vi "CRYGet Scale Format Info.vi"(11 "FormatString":string) -> (3 "ScaleFormat":T1)   [LabVIEW 2013]
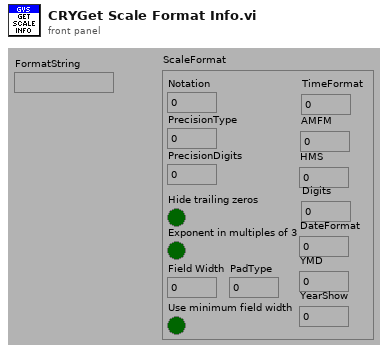
[diagram p1: front panel]
types:
  T1 = cluster{"Notation":i32, "PrecisionType":u16, "PrecisionDigits":u16, "Hide trailing zeros":bool, "Exponent in multiples of 3":bool, "Field Width":u16, "PadType":u16, "Use minimum field width":bool, "TimeFormat":u16, "AMFM":u16, "HMS":u16, "Digits":u16, "DateFormat":u16, "YMD":u16, "YearShow":u16}
  T2 = enum16{"OK", "Yes", "YesNo", "YesNoCancel", "ReplaceAppend"}
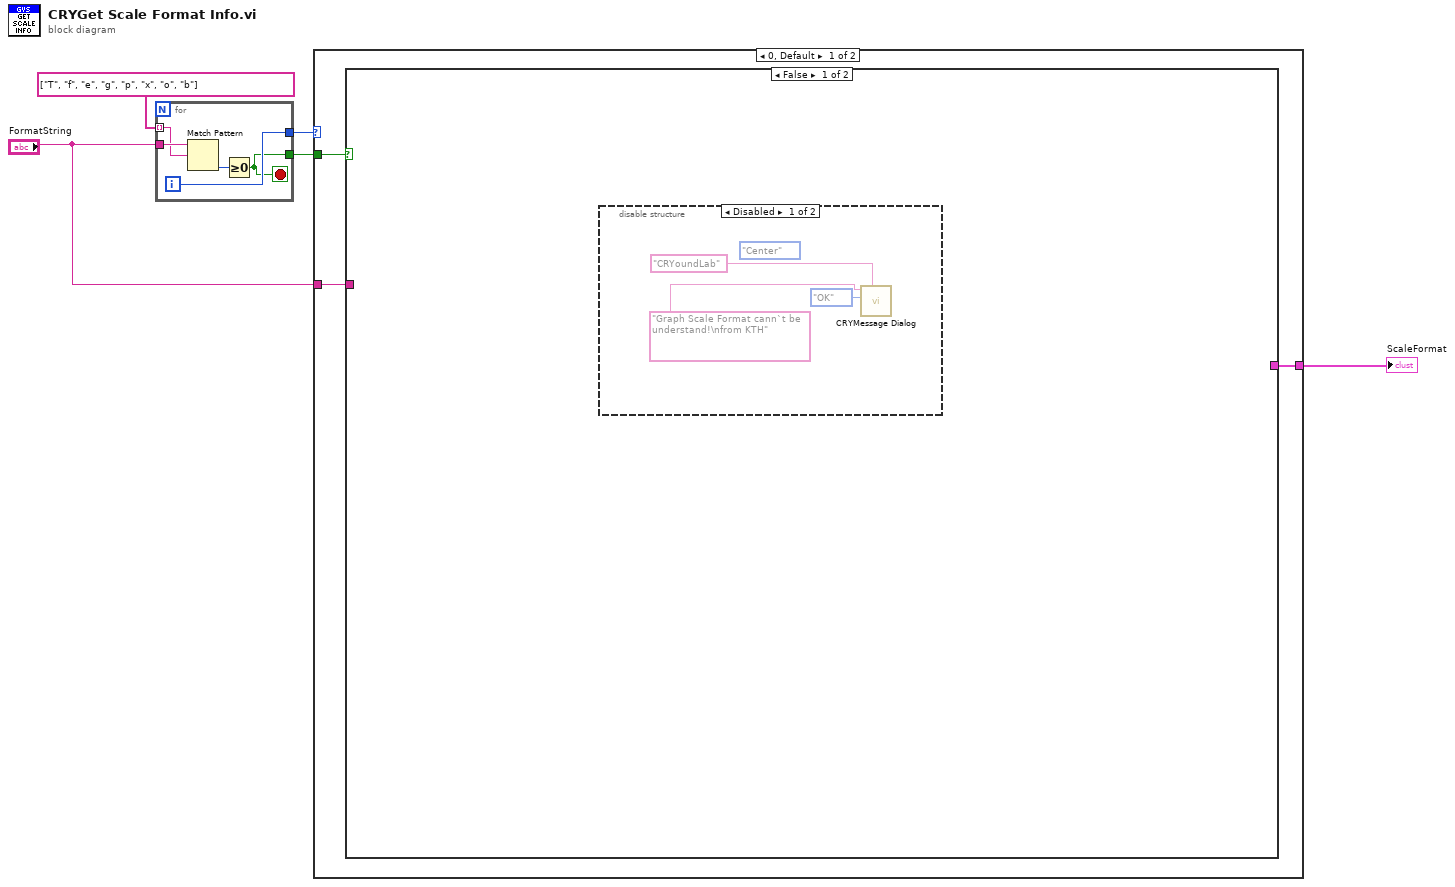
[diagram p0: block diagram]
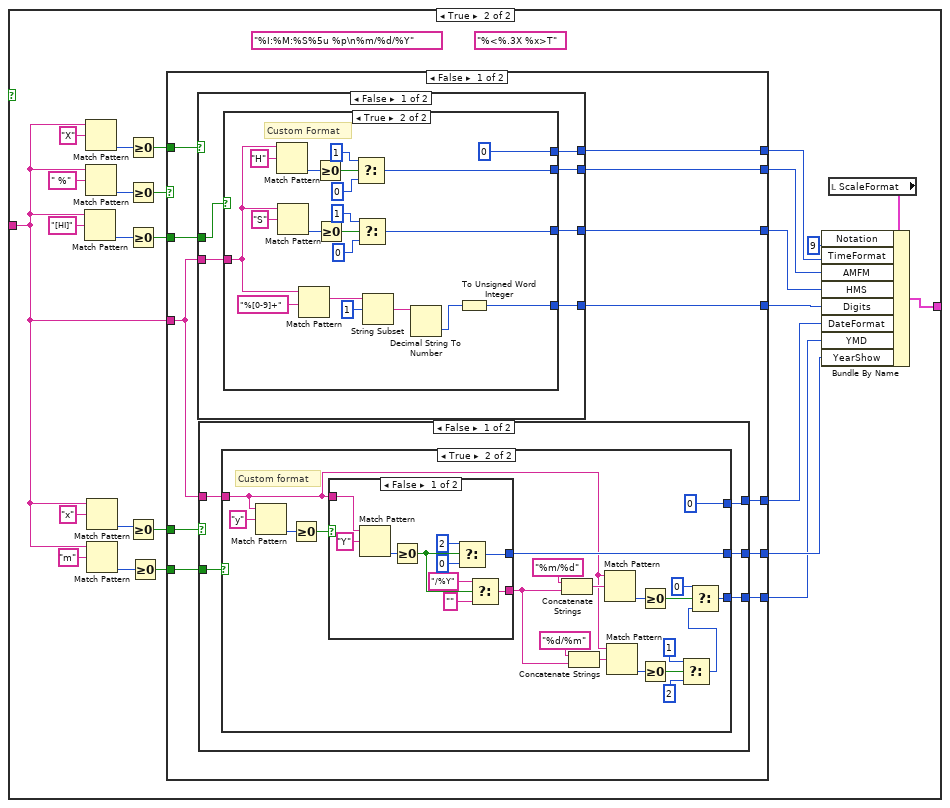
[diagram p3: hidden frame]
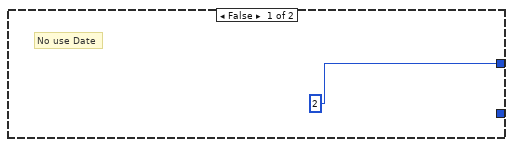
[diagram p4: hidden frame]
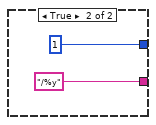
[diagram p5: hidden frame]
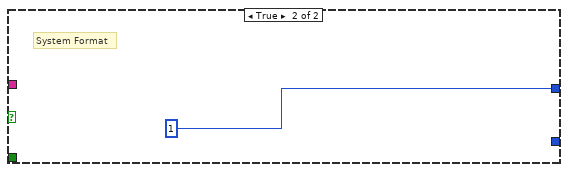
[diagram p6: hidden frame]
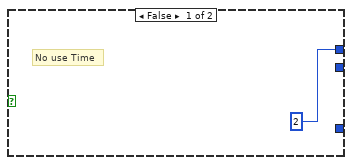
[diagram p7: hidden frame]
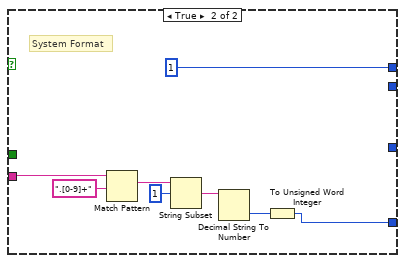
[diagram p8: hidden frame]
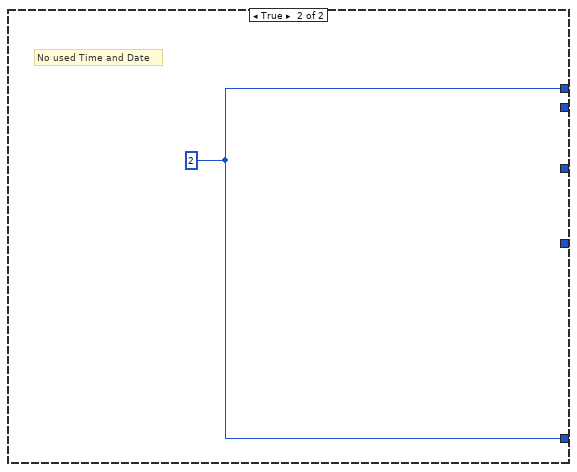
[diagram p9: hidden frame]
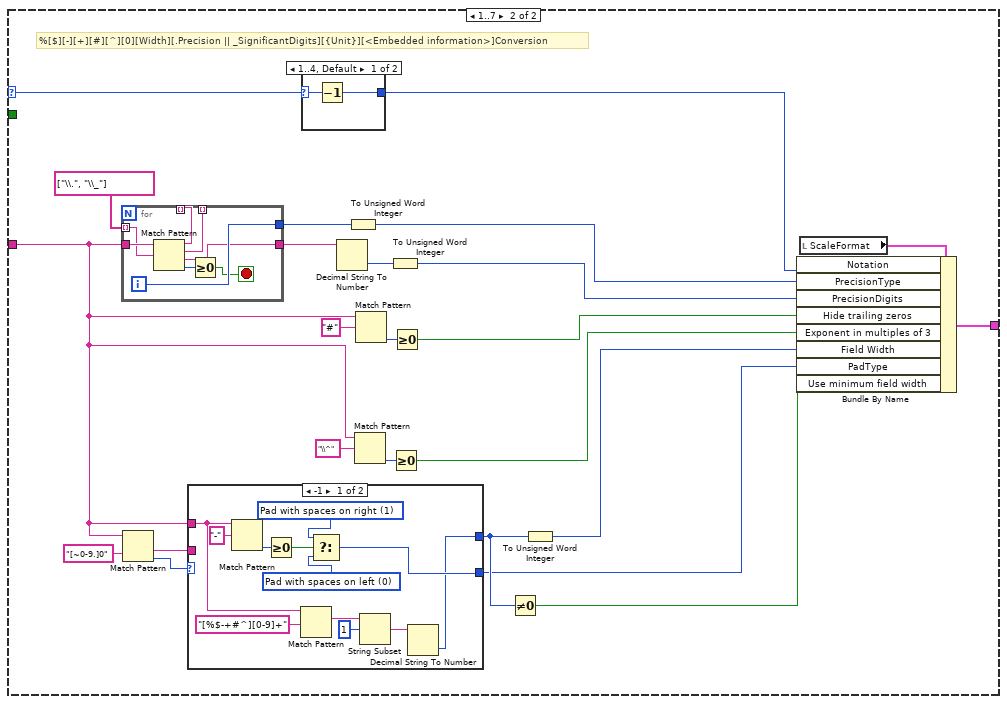
[diagram p10: hidden frame]
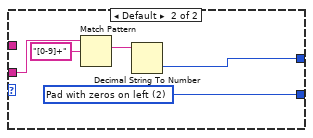
[diagram p12: hidden frame]
diagram:
  n1 = for {
    tunnel: "FormatString" -> [w9]
    tunnel: string[] ["T", "f", "e", "g", "p", "x", "o", "b"] -> [w8] mode=indexing
    tunnel: [w7] -> w2
    tunnel: [w6] -> w1
    i -> [w7]
    stop <- w6 stop-if-true
    n2 = Match Pattern(string=w9, regular expression=w8) -> (offset past match=w10:i32)  [unwired: 1 in, 3 out]
    n3 = Greater Or Equal To 0?(x=w10) -> (x >= 0?=w6:bool)
  }
  n4 = case shown="0, Default" w2 {
    selector: w2 -> [_ w130]
    tunnel: "FormatString" -> [w12 w143]
    tunnel: [w11 w139] -> w3
    tunnel: w1 -> [w13 _]
    frame 0, Default {
      n5 = case shown="False" w13 {
        tunnel: w12 -> [_ w23]
        tunnel: [_ w37] -> w11
        frame False {
          n6 = disable-structure shown="Disabled" {
            frame Disabled {
              (unwired) enum16{"Left", "Center", "Right"}."Center" ("Justify Message (Left)")
              n7 = call "CRYMessage Dialog.vi"("Window Title"="CRYoundLab" ("Window Title (\"\")"), "YesNoCancel"=T2."OK", "Message Content"="Graph Scale Format cann`t be understand!\nfrom KTH" ("message")) -> ()  [unwired: 7 in, 2 out]
            }
            frame Enabled {
            }
          }
        }
        frame True {
          (unwired) "%<%.3X %x>T" ("format string")
          (unwired) "%I:%M:%S%5u %p\n%m/%d/%Y" ("format string")
          n8 = Match Pattern(string=w23, regular expression="[HI]") -> (offset past match=w28:i32)  [unwired: 1 in, 3 out]
          n9 = Match Pattern(string=w23, regular expression="X") -> (offset past match=w40:i32)  [unwired: 1 in, 3 out]
          n10 = Match Pattern(string=w23, regular expression=" %") -> (offset past match=w31:i32)  [unwired: 1 in, 3 out]
          n11 = Match Pattern(string=w23, regular expression="x") -> (offset past match=w39:i32)  [unwired: 1 in, 3 out]
          n12 = Match Pattern(string=w23, regular expression="m") -> (offset past match=w27:i32)  [unwired: 1 in, 3 out]
          n13 = Greater Or Equal To 0?(x=w40) -> (x >= 0?=w36:bool)
          n14 = Greater Or Equal To 0?(x=w31) -> (x >= 0?=w30:bool)
          n15 = Greater Or Equal To 0?(x=w28) -> (x >= 0?=w24:bool)
          n16 = Greater Or Equal To 0?(x=w39) -> (x >= 0?=w34:bool)
          n17 = Greater Or Equal To 0?(x=w27) -> (x >= 0?=w25:bool)
          n18 = case shown="False" w30 {
            tunnel: w36 -> [w54 _]
            tunnel: [w53 w129] -> w35
            tunnel: w34 -> [w52 _]
            tunnel: [w51 w129] -> w33
            tunnel: w25 -> [w50 _]
            tunnel: w24 -> [w49 _]
            tunnel: w23 -> [w45 _]
            tunnel: [w48 _] -> w22
            tunnel: [w47 _] -> w21
            tunnel: [w46 _] -> w20
            tunnel: [w44 _] -> w19
            tunnel: [w43 _] -> w18
            frame False {
              n19 = case shown="False" w54 {
                tunnel: [w98 u16 1 ("TimeFormat")] -> w53
                tunnel: w49 -> [w99 _]
                tunnel: w45 -> [w97 w122]
                tunnel: [w96 _] -> w48
                tunnel: [w95 _] -> w47
                tunnel: [w94 w121] -> w46
                frame False {
                  n20 = case shown="True" w99 {
                    tunnel: [u16 2 ("TimeFormat") u16 0 ("TimeFormat")] -> w98
                    tunnel: w97 -> [_ w106]
                    tunnel: [_ w114] -> w96
                    tunnel: [_ w108] -> w95
                    tunnel: [_ w101] -> w94
                    frame False {
                      # "No use Time"
                    }
                    frame True {
                      # "Custom Format"
                      n21 = Match Pattern(string=w106, regular expression="H") -> (offset past match=w118:i32)  [unwired: 1 in, 3 out]
                      n22 = Match Pattern(string=w106, regular expression="S") -> (offset past match=w110:i32)  [unwired: 1 in, 3 out]
                      n23 = Match Pattern(string=w106, regular expression="%[0-9]+") -> (match substring=w105:string)  [unwired: 1 in, 3 out]
                      n24 = Greater Or Equal To 0?(x=w118) -> (x >= 0?=w117:bool)
                      n25 = Greater Or Equal To 0?(x=w110) -> (x >= 0?=w111:bool)
                      n26 = Select(t=u16 1 ("TimeFormat"), s=w117, f=u16 0 ("TimeFormat")) -> (s? t:f=w114:u16)
                      n27 = Select(t=u16 1 ("TimeFormat"), s=w111, f=u16 0 ("TimeFormat")) -> (s? t:f=w108:u16)
                      n28 = String Subset(string=w105, offset (0)=1) -> (substring=w103:string)  [unwired: 1 in]
                      n29 = Decimal String To Number(string=w103) -> (number=w102:i32)  [unwired: 2 in, 1 out]
                      n30 = To Unsigned Word Integer(number=w102) -> (unsigned 16bit integer=w101:u16)
                    }
                  }
                }
                frame True {
                  # "System Format"
                  n31 = Match Pattern(string=w122, regular expression=".[0-9]+") -> (match substring=w126:string)  [unwired: 1 in, 3 out]
                  n32 = String Subset(string=w126, offset (0)=1) -> (substring=w124:string)  [unwired: 1 in]
                  n33 = Decimal String To Number(string=w124) -> (number=w123:i32)  [unwired: 2 in, 1 out]
                  n34 = To Unsigned Word Integer(number=w123) -> (unsigned 16bit integer=w121:u16)
                }
              }
              n35 = case shown="False" w52 {
                tunnel: [w58 u16 1 ("TimeFormat")] -> w51
                tunnel: w50 -> [w59 _]
                tunnel: w45 -> [w57 _]
                tunnel: [w56 _] -> w44
                tunnel: [w55 _] -> w43
                frame False {
                  n36 = case shown="True" w59 {
                    tunnel: [u16 2 ("TimeFormat") u16 0 ("TimeFormat")] -> w58
                    tunnel: w57 -> [_ w61]
                    tunnel: [_ w76] -> w56
                    tunnel: [_ w62] -> w55
                    frame False {
                      # "No use Date"
                    }
                    frame True {
                      # "Custom format"
                      n37 = Match Pattern(string=w61, regular expression="y") -> (offset past match=w78:i32)  [unwired: 1 in, 3 out]
                      n38 = Greater Or Equal To 0?(x=w78) -> (x >= 0?=w77:bool)
                      n39 = case shown="False" w77 {
                        tunnel: [w85 u16 1 ("TimeFormat")] -> w76
                        tunnel: w61 -> [w88 _]
                        tunnel: [w82 "/%y" ("FormatString")] -> w69
                        frame False {
                          n40 = Match Pattern(string=w88, regular expression="Y") -> (offset past match=w90:i32)  [unwired: 1 in, 3 out]
                          n41 = Greater Or Equal To 0?(x=w90) -> (x >= 0?=w84:bool)
                          n42 = Select(t=u16 2 ("TimeFormat"), s=w84, f=u16 0 ("TimeFormat")) -> (s? t:f=w85:u16)
                          n43 = Select(t="/%Y" ("regular expression"), s=w84, f="" ("regular expression")) -> (s? t:f=w82:string)
                        }
                        frame True {
                        }
                      }
                      n44 = Concatenate Strings("%m/%d" ("regular expression"), w69) -> (w73:string)
                      n45 = Concatenate Strings("%d/%m" ("regular expression"), w69) -> (w72:string)
                      n46 = Match Pattern(string=w61, regular expression=w73) -> (offset past match=w75:i32)  [unwired: 1 in, 3 out]
                      n47 = Match Pattern(string=w61, regular expression=w72) -> (offset past match=w70:i32)  [unwired: 1 in, 3 out]
                      n48 = Greater Or Equal To 0?(x=w75) -> (x >= 0?=w68:bool)
                      n49 = Greater Or Equal To 0?(x=w70) -> (x >= 0?=w65:bool)
                      n50 = Select(t=u16 1 ("TimeFormat"), s=w65, f=u16 2 ("TimeFormat")) -> (s? t:f=w63:u16)
                      n51 = Select(t=u16 0 ("TimeFormat"), s=w68, f=w63) -> (s? t:f=w62:u16)
                    }
                  }
                }
                frame True {
                  # "System Format"
                }
              }
            }
            frame True {
              w129 = u16 2 ("TimeFormat")
              # "No used Time and Date"
            }
          }
          n52 = local read "ScaleFormat"() -> (w38:T1)
          n53 = Bundle By Name(cluster=w38, "Notation"=9, "TimeFormat"=w35, "AMFM"=w22, "HMS"=w21, "Digits"=w20, "DateFormat"=w33, "YMD"=w18, "YearShow"=w19) -> (w37:T1)
        }
      }
    }
    frame 1..7 {
      # "%[$][-][+][#][^][0][Width][.Precision || _SignificantDigits][{Unit}][<Embedded information>]Conversion"
      n54 = for {
        tunnel: w143 -> [w180]
        tunnel: string[] ["\\.", "\\_"] -> [w179] mode=indexing
        tunnel: [w178] -> w152
        tunnel: [w177] -> w151
        tunnel: [w175] -> _ mode=indexing
        tunnel: [w174] -> _ mode=indexing
        i -> [w178]
        stop <- w176 stop-if-true
        n55 = Match Pattern(string=w180, regular expression=w179) -> (before substring=w175:string, match substring=w174:string, after substring=w177:string, offset past match=w181:i32)  [unwired: 1 in]
        n56 = Greater Or Equal To 0?(x=w181) -> (x >= 0?=w176:bool)
      }
      n57 = Match Pattern(string=w143, regular expression="[~0-9.]0") -> (after substring=w147:string, offset past match=w146:i32)  [unwired: 1 in, 2 out]
      n58 = case shown="-1" w146 {
        tunnel: w147 -> [_ w171]
        tunnel: w143 -> [w162 _]
        tunnel: [w163 w170] -> w133
        tunnel: [w157 w169] -> w141
        frame -1 {
          w164 = u16 0 items=["Pad with spaces on left", "Pad with spaces on right", "Pad with zeros on left"] ("PadType")
          w165 = u16 1 items=["Pad with spaces on left", "Pad with spaces on right", "Pad with zeros on left"] ("PadType")
          n59 = Match Pattern(string=w162, regular expression="-" ("format string")) -> (offset past match=w168:i32)  [unwired: 1 in, 3 out]
          n60 = Greater Or Equal To 0?(x=w168) -> (x >= 0?=w166:bool)
          n61 = Match Pattern(string=w162, regular expression="[%$-+#^][0-9]+") -> (match substring=w159:string)  [unwired: 1 in, 3 out]
          n62 = Select(t=w165, s=w166, f=w164) -> (s? t:f=w163:u16)
          n63 = String Subset(string=w159, offset (0)=1) -> (substring=w158:string)  [unwired: 1 in]
          n64 = Decimal String To Number(string=w158) -> (number=w157:i32)  [unwired: 2 in, 1 out]
        }
        frame Default {
          w170 = u16 2 items=["Pad with spaces on left", "Pad with spaces on right", "Pad with zeros on left"] ("PadType")
          n65 = Match Pattern(string=w171, regular expression="[0-9]+") -> (match substring=w172:string)  [unwired: 1 in, 3 out]
          n66 = Decimal String To Number(string=w172) -> (number=w169:i32)  [unwired: 2 in, 1 out]
        }
      }
      n67 = case shown="1..4, Default" w130 {
        selector: w130 -> [w155 w156]
        tunnel: [w154 w156] -> w138
        frame 1..4, Default {
          n68 = Decrement(x=w155) -> (x-1=w154:i32)
        }
        frame 5..7 {
        }
      }
      n69 = Decimal String To Number(string=w151) -> (number=w142:i32)  [unwired: 2 in, 1 out]
      n70 = To Unsigned Word Integer(number=w152) -> (unsigned 16bit integer=w137:u16)
      n71 = Match Pattern(string=w143, regular expression="\\^" ("format string")) -> (offset past match=w150:i32)  [unwired: 1 in, 3 out]
      n72 = Match Pattern(string=w143, regular expression="#" ("format string")) -> (offset past match=w144:i32)  [unwired: 1 in, 3 out]
      n73 = To Unsigned Word Integer(number=w142) -> (unsigned 16bit integer=w136:u16)
      n74 = Greater Or Equal To 0?(x=w150) -> (x >= 0?=w134:bool)
      n75 = Greater Or Equal To 0?(x=w144) -> (x >= 0?=w135:bool)
      n76 = Not Equal To 0?(x=w141) -> (x != 0?=w131:bool)
      n77 = To Unsigned Word Integer(number=w141) -> (unsigned 16bit integer=w132:u16)
      n78 = local read "ScaleFormat"() -> (w140:T1)
      n79 = Bundle By Name(cluster=w140, "Notation"=w138, "PrecisionType"=w137, "PrecisionDigits"=w136, "Hide trailing zeros"=w135, "Exponent in multiples of 3"=w134, "Field Width"=w132, "PadType"=w133, "Use minimum field width"=w131) -> (w139:T1)
    }
  }
  "ScaleFormat" <- w3
